vi "PH_Beamline_Chief.Settings 2 Data String.vi"(1 "Settings":T1) -> (0 "Data String":string)   [LabVIEW 2014, in "PH_Beamline_Chief.lvlib"]
uses:
  PH_Beamline_Chief.lvlib
  PH_Beamline_Chief.Settings.ctl
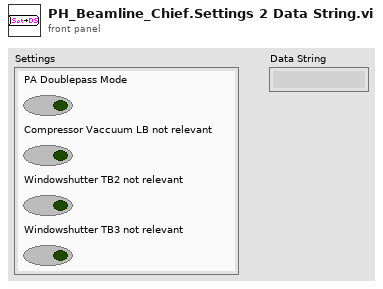
[diagram p1: front panel]
types:
  T1 = typedef "PH_Beamline_Chief.lvlib/PH_Beamline_Chief.Settings.ctl" = cluster{"PA Doublepass Mode":bool, "Compressor Vaccuum LB not relevant":bool, "Windowshutter TB2 not relevant":bool, "Windowshutter TB3 not relevant":bool}
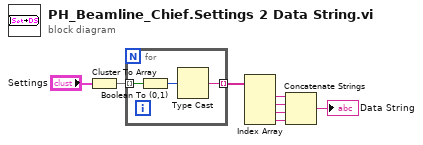
[diagram p0: block diagram]
diagram:
  n1 = Cluster To Array(cluster="Settings") -> (array=w7:bool[])
  n2 = for {
    tunnel: [w11] -> w6 mode=indexing
    tunnel: w7 -> [w10] mode=indexing
    n3 = Boolean To (0,1)(Boolean=w10) -> (0, 1=w9:i16)
    n4 = Type Cast(x=w9) -> (*(type *) &x=w11:string)  [unwired: 1 in]
  }
  n5 = Index Array(array=w6) -> (element #1=w5:string, element #2=w4:string, element #3=w3:string, element #4=w2:string)  [unwired: 4 in]
  n6 = Concatenate Strings(w5, w4, w3, w2) -> (→"Data String":string)
